vi "finishup.vi"(8 "error in (no error)":errorcluster, 11 "ActionEditor in":refnum<class "ActionEditor.lvclass">) -> (0 "error out":errorcluster, 3 "ActionEditor out":refnum<class "ActionEditor.lvclass">)   [LabVIEW 2009, in "Views.lvlib" / "ScriptEditor.lvlib" / "ActionEditor.lvclass"]
uses:
  ActionEditor.lvclass
  ActionEditor.lvclass/ActionEditor.ctl
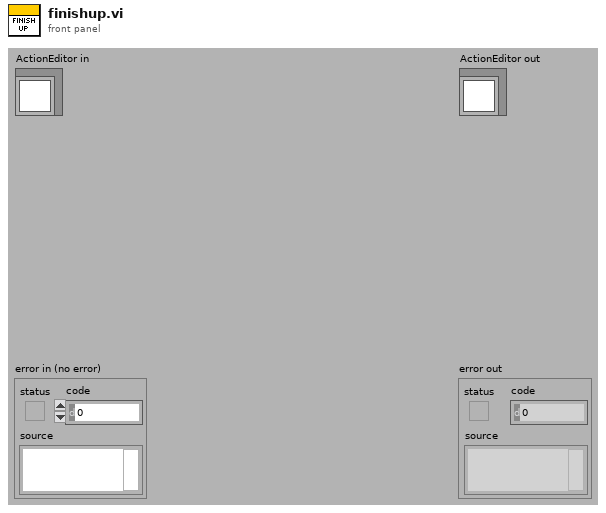
[diagram p1: front panel]
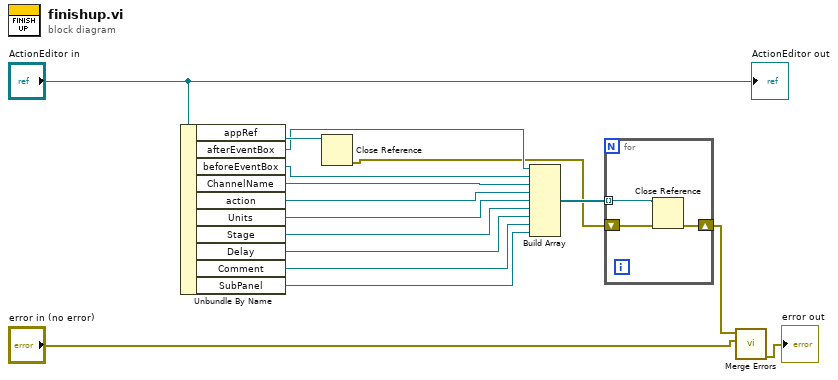
[diagram p0: block diagram]
diagram:
  n1 = Unbundle By Name("ActionEditor in") -> ("appRef"=w15:refnum<vi>, "afterEventBox"=w7:refnum<vi>, "beforeEventBox"=w6:refnum<vi>, "ChannelName"=w14:refnum<vi>, "action"=w13:refnum<vi>, "Units"=w12:refnum<vi>, "Stage"=w11:refnum<vi>, "Delay"=w10:refnum<vi>, "Comment"=w9:refnum<vi>, "SubPanel"=w8:refnum<vi>)
  n2 = Close Reference(reference=w15) -> (error out=w1:errorcluster)  [unwired: 1 in]
  n3 = Build Array(w7, w6, w14, w13, w12, w11, w10, w9, w8) -> (w5:refnum<vi>[])
  n4 = for {
    tunnel: w5 -> [w19] mode=indexing
    shift-right: [w17] -> w3
    shift-left: w1 -> [w18]
    n5 = Close Reference(reference=w19, error in (no error)=w18) -> (error out=w17:errorcluster)
  }
  n6 = call <vilib>:"Merge Errors.vi"("error in 2 (no error)"="error in (no error)", "error in 1 (no error)"=w3) -> ("error out"=→"error out":errorcluster)  [unwired: 5 in]
  "ActionEditor out" <- "ActionEditor in"
